vi "Replace Tag with Array for CSM Script.vi"(8 "Error in":errorcluster caption="Error in (no error)", 9 "Enum":enum16{"<1>", "<2>", "<3>", "<4>"}(ring), 10 "replace string":string[](array[string]), 11 "single-line text":string="All Data Saved@TDMS >> API: Terminate@<1> -><register>") -> (0 "Error out":errorcluster, 3 "States":string)   [LabVIEW 2017]
uses:
  Communicable State Machine.lvlib
panel:
  # "Connector Pane"
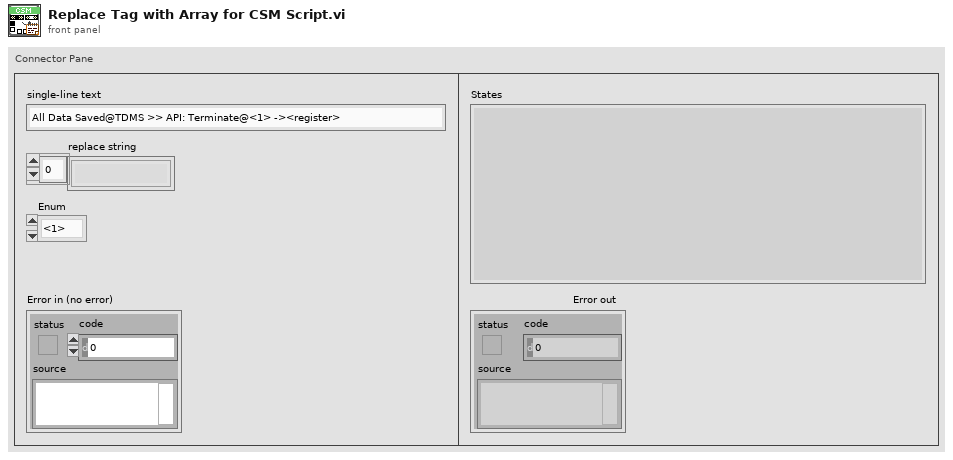
[diagram p1: front panel]
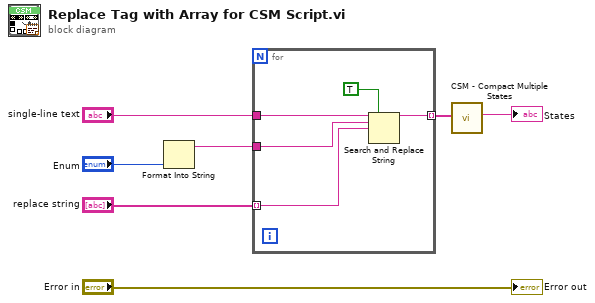
[diagram p0: block diagram]
diagram:
  n1 = Format Into String("Enum") -> (resulting string=w1:string)  [unwired: 3 in, 1 out]
  n2 = for {
    tunnel: "single-line text" -> [w12]
    tunnel: "replace string" -> [w10] mode=indexing
    tunnel: [w9] -> w6 mode=indexing
    tunnel: w1 -> [w8]
    n3 = Search and Replace String(replace all?=TRUE ("replace all? (F)"), input string=w12, search string=w8, replace string=w10) -> (result string=w9:string)  [unwired: 4 in, 3 out]
  }
  n4 = call "CSM - Compact Multiple States.vi"("Multiple States"=w6) -> ("States"=→"States":string)  [unwired: 9 in]
  "Error out" <- "Error in"
